vi "GPIB_findInstrument.vi"(9 "ID command":string, 10 "revised Instrument address":refnum<visa-resource-name>, 11 "Instrument name IN":string) -> (2 "revised GPIB address OUT":refnum<visa-resource-name>)   [LabVIEW 2019, in "InstrControl.lvclass"]
uses:
  InstrControl.lvclass
panel:
  in  "Refresh Button":bool
  in  "Cancel":bool
  in  "OK":bool
  out "instrument responses":string[](array[string])
  out "instrument addresses found":string[](array[string])
  out "error out":errorcluster
  in  "error in (no error)":errorcluster
  # "Find GPIB instrument:"
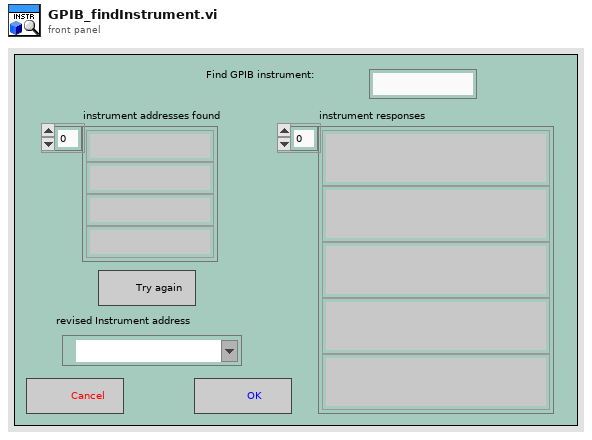
[diagram p1: front panel]
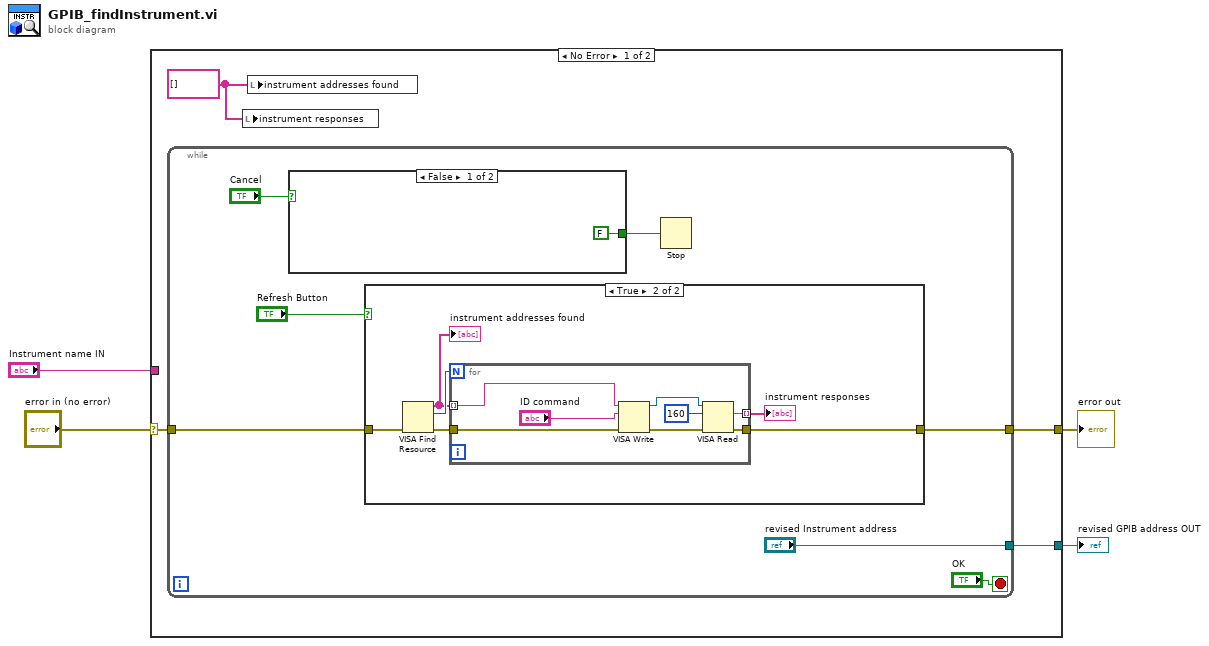
[diagram p0: block diagram]
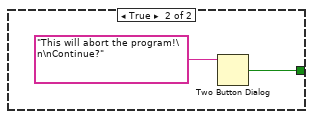
[diagram p3: hidden frame]
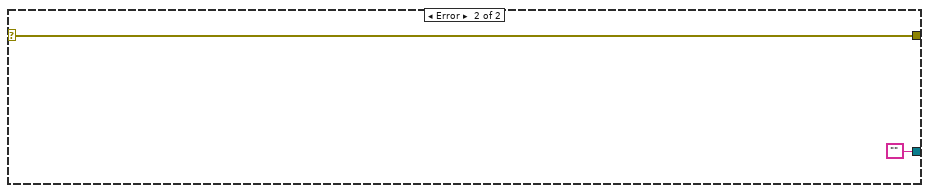
[diagram p4: hidden frame]
diagram:
  n1 = case shown="No Error" "error in (no error)" {
    selector: "error in (no error)" -> [w8 w35]
    tunnel: [w7 w35] -> w3
    tunnel: [w6 ""] -> w2
    tunnel: "Instrument name IN" -> [_ _]
    frame No Error {
      w5 = string[] []
      n2 = while {
        tunnel: w8 -> [w15]
        tunnel: [w11] -> w7
        tunnel: ["revised Instrument address"] -> w6
        stop <- "OK" stop-if-true
        n3 = case shown="False" "Cancel" {
          tunnel: [FALSE w32] -> w13
          frame False {
          }
          frame True {
            n4 = Two Button Dialog(message="This will abort the program!\n\nContinue?") -> (T button?=w32:bool)  [unwired: 2 in]
          }
        }
        n5 = case shown="True" "Refresh Button" {
          tunnel: w15 -> [w16 w20]
          tunnel: [w16 w17] -> w11
          frame False {
          }
          frame True {
            n6 = VISA Find Resource(8:w20) -> (0:w22:errorcluster, 2:w21:u32, 3:w19:string[])  [unwired: 2 in]
            "instrument addresses found" <- w19
            n7 = for {
              N: w21 -> [_]
              tunnel: w19 -> [w25] mode=indexing
              tunnel: w22 -> [w23]
              tunnel: [w27] -> w17
              tunnel: [w26] -> w18 mode=indexing
              n8 = VISA Write(VISA resource name=w25, write buffer="ID command", error in (no error)=w23) -> (VISA resource name out=w29:refnum<visa-resource-name>, error out=w28:errorcluster)  [unwired: 1 out]
              n9 = VISA Read(VISA resource name=w29, byte count=160, error in (no error)=w28) -> (read buffer=w26:string, error out=w27:errorcluster)  [unwired: 2 out]
            }
            "instrument responses" <- w18
          }
        }
        n10 = Stop(stop? (T)=w13) -> ()
      }
      n11 = local write "instrument responses"(w5) -> ()
      n12 = local write "instrument addresses found"(w5) -> ()
    }
    frame Error {
    }
  }
  "error out" <- w3
  "revised GPIB address OUT" <- w2
